vi "Swap (No Check).vi"(8 "error in (no error)":errorcluster, 9 "size":u64 format="%d bytes", 10 "Pointer b":refnum<class "Pointer.lvclass">, 11 "Pointer a":refnum<class "Pointer.lvclass">) -> (0 "error out":errorcluster, 2 "Pointer b":refnum<class "Pointer.lvclass">, 3 "Pointer a":refnum<class "Pointer.lvclass">)   [LabVIEW 2016, in "Memory Manager.lvlib" / "Pointer.lvclass"]
doc: "Swaps <b>size</b> bytes between the section of memory referred to by the two provided <b>pointers</b>. The source and destination memory blocks should not overlap.\n\n<b>Note:</b> This VI is <b>unsafe</b>.\n\nUnsafe means that this function does not evaluate the size parameter of <b>pointer a</b> and <b>pointer b</b> before peforming a memory read/write. Reading/writing more data to a pointer than it has allocated can corrupt or crash LabVIEW."
uses:
  Pointer.lvclass
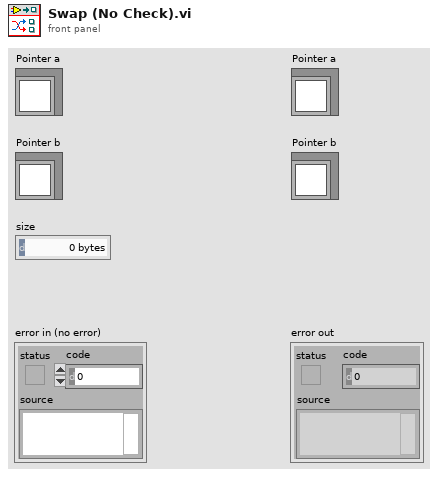
[diagram p1: front panel]
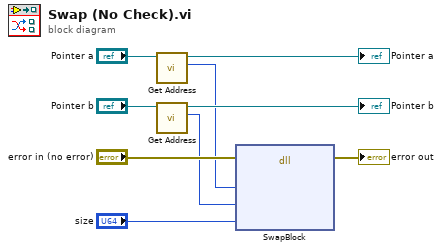
[diagram p0: block diagram]
diagram:
  n1 = call "Get Address.vi"("Pointer in"="Pointer a") -> ("address"=w3:u64, "Pointer out"=→"Pointer a":refnum<class "Pointer.lvclass">)  [unwired: 9 in]
  n2 = call "Get Address.vi"("Pointer in"="Pointer b") -> ("address"=w2:u64, "Pointer out"=→"Pointer b":refnum<class "Pointer.lvclass">)  [unwired: 9 in]
  n3 = dll-call lib="LabVIEW" fn="SwapBlock"(error in="error in (no error)", "src"=w3, "dst"=w2, "size"="size") -> (error out=→"error out":errorcluster)  [unwired: 6 in, 1 out]
